vi "Set Line Width.vi"(8 "error in (no error)":errorcluster, 9 "width":u8, 10 "Channel":i32, 11 "Graph Manager in":refnum<class "Graph Manager.lvclass">) -> (0 "error out":errorcluster, 2 "Channel out":i32, 3 "Graph Manager out":refnum<class "Graph Manager.lvclass">)   [LabVIEW 2016, in "Graph Manager.lvclass"]
uses:
  Graph Manager.lvclass
  Graph Manager.lvclass/Graph Manager.ctl
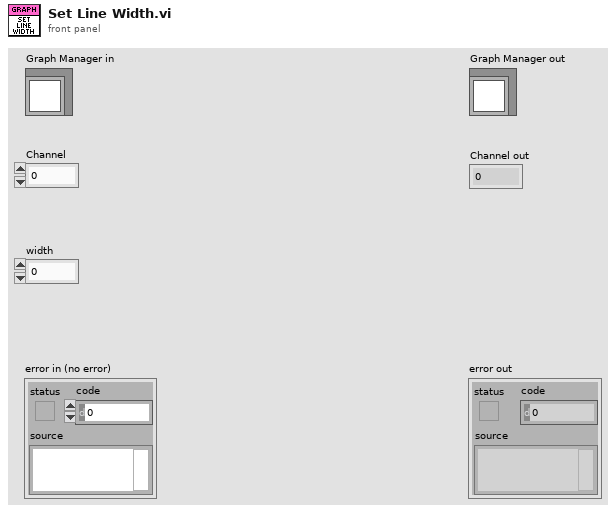
[diagram p1: front panel]
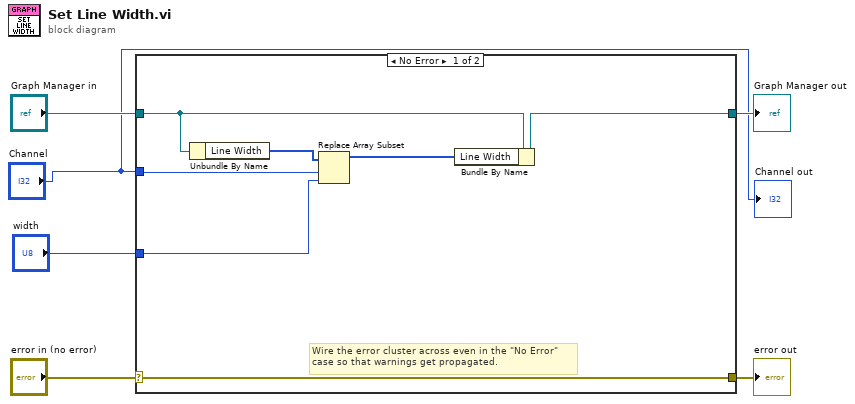
[diagram p0: block diagram]
diagram:
  n1 = case shown="No Error" "error in (no error)" {
    selector: "error in (no error)" -> [w13 w15]
    tunnel: [w13 w15] -> w5
    tunnel: [w10 w14] -> w3
    tunnel: "Graph Manager in" -> [w11 w14]
    tunnel: "width" -> [w8 _]
    tunnel: "Channel" -> [w7 _]
    frame No Error {
      # "Wire the error cluster across even in the \"No Error\"\ncase so that warnings get propagated."
      n2 = Unbundle By Name(w11) -> ("Line Width"=w12:u8[])
      n3 = Replace Array Subset(array=w12, new element=w8, index=w7) -> (w9:u8[])
      n4 = Bundle By Name(cluster=w11, "Line Width"=w9) -> (w10:refnum<class "Graph Manager.lvclass">)
    }
    frame Error {
    }
  }
  "error out" <- w5
  "Graph Manager out" <- w3
  "Channel out" <- "Channel"
